vi "AutoIntakeFront_new.vi"() -> ()   [LabVIEW 2015]
uses:
  IntakeController/Typedef/Command List.ctl
  Typedef/IntakeControllerActions.ctl
  IntakeController/Typedef/Front Arm List.ctl
  IntakeController/Typedef/Rear Arm List.ctl
  Front Arm Positions.vi
  IntakeController/SubVI/GetIntakeQueue.vi
panel:
  in  "Command List":T1=[{"Cmd"=enum."Set Roller Front", "Value"=0.8, "Front Arm"=enum."Down", "Rear Arm"=enum."Down"}, {"Cmd"=enum."Go To Angle Front", "Value"=0.0, "Front Arm"=enum."Pickup", "Rear Arm"=enum."Down"}, {"Cmd"=enum."Go To Angle Rear", "Value"=0.0, "Front Arm"=enum."Down", "Rear Arm"=enum."Intake Block"}, {"Cmd"=enum."Wait ms", "Value"=600.0, "Front Arm"=enum."Down", "Rear Arm"=enum."Down"}, {"Cmd"=enum."Wait on Intake Front", "Value"=0.0, "Front Arm"=enum."Down", "Rear Arm"=enum."Down"}, {"Cmd"=enum."Wait ms", "Value"=100.0, "Front Arm"=enum."Down", "Rear Arm"=enum."Down"}, {"Cmd"=enum."Set Roller Front", "Value"=0.0, "Front Arm"=enum."Down", "Rear Arm"=enum."Down"}, {"Cmd"=enum."Go To Angle Front", "Value"=0.0, "Front Arm"=enum."Turtle", "Rear Arm"=enum."Down"}, {"Cmd"=enum."Wait ms", "Value"=1000.0, "Front Arm"=enum."Down", "Rear Arm"=enum."Turtle"}, {"Cmd"=enum."Go To Angle Rear", "Value"=0.0, "Front Arm"=enum."Down", "Rear Arm"=enum."Turtle"}]
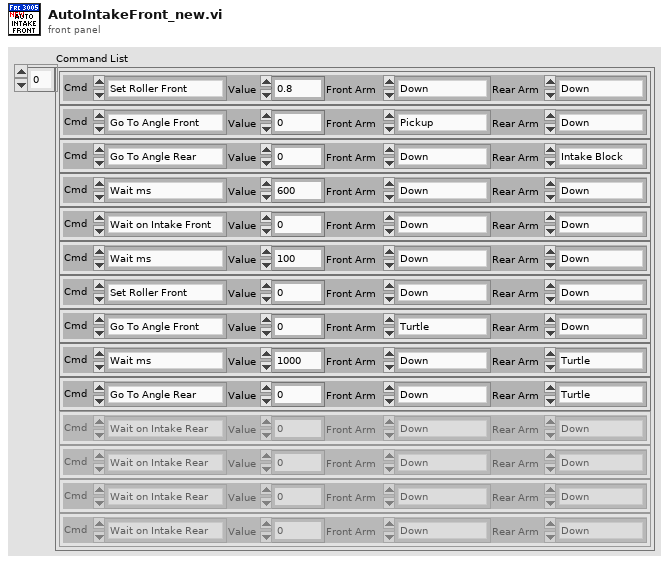
[diagram p1: front panel]
types:
  T1 = typedef "Command List.ctl" = cluster{"Cmd":T2, "Value":dbl, "Front Arm":T3, "Rear Arm":T4}[]
  T2 = typedef "IntakeControllerActions.ctl" = enum16{"Wait on Intake Rear", "Wait on Angle Rear", "Go To Angle Rear", "Wait on Intake Front", "Wait on Angle Front", "Set Roller Front", "Set Roller Rear", "Go To Angle Front", "Wait ms"}
  T3 = typedef "Front Arm List.ctl" = enum16{"Down", "Pickup", "Shoot", "Turtle", "Intake Transfer", "Extra1", "Extra2"}
  T4 = typedef "Rear Arm List.ctl" = enum16{"Down", "Pickup", "Shoot", "Turtle", "Intake Block", "Intake Transfer", "Extra1", "Extra2"}
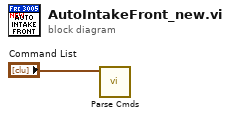
[diagram p0: block diagram]
diagram:
  n1 = call "Parse Cmds.vi"("Command List"="Command List") -> ()  [unwired: 11 in]
